vi "Terminal-Alert-6133.vi"(10 "检验次数（5）":i32=5, 11 "6133":T1) -> (3 "6133输出":T1)   [LabVIEW 2014]
uses:
  Terminal-Global-ReferenceValues.vi
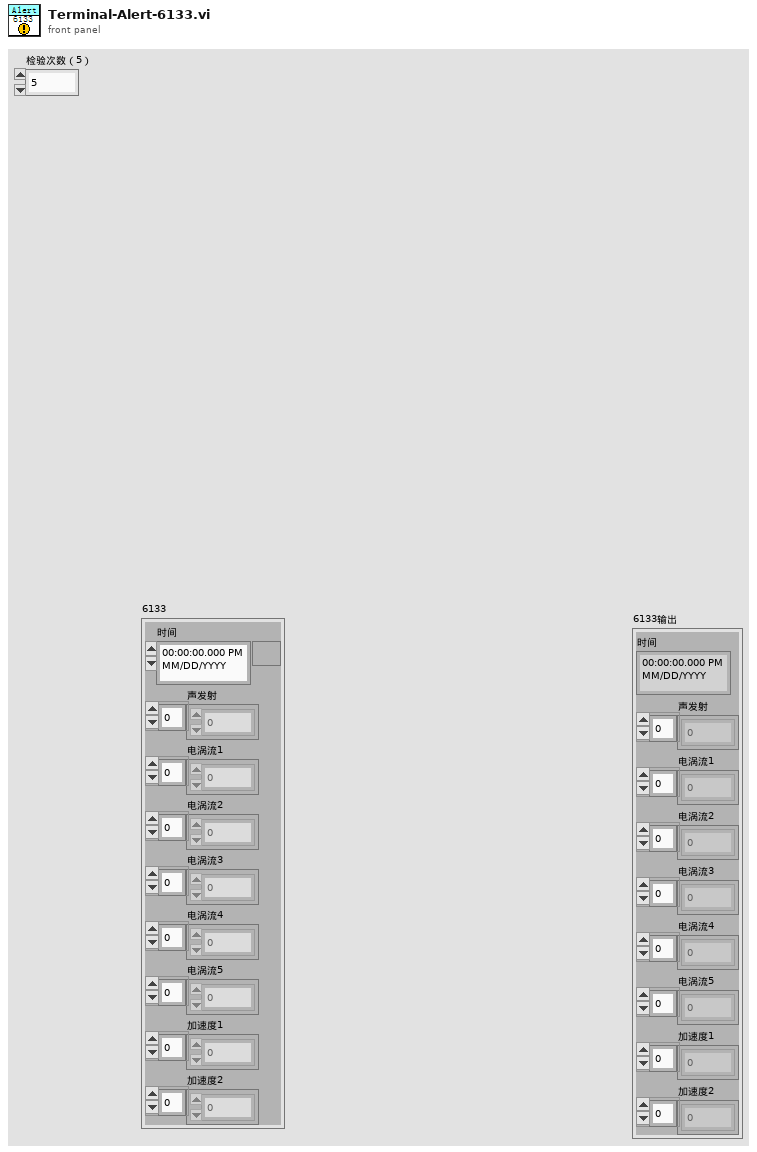
[diagram p1: front panel]
types:
  T1 = cluster{"时间":timestamp, "声发射":sgl[], "电涡流1":sgl[], "电涡流2":sgl[], "电涡流3":sgl[], "电涡流4":sgl[], "电涡流5":sgl[], "加速度1":sgl[], "加速度2":sgl[]}
  T2 = cluster{"试验ID":u32, "报警级别":string, "报警系统":string, "报警详情":string, "备注":string}
  T3 = cluster{"陪试轴承润滑单元":cluster{"出油温度T1":dbl, "出油温度T2":dbl}, "试验轴承润滑单元":cluster{"外壳振动1，A1":dbl, "外壳振动2，A2":dbl, "轴承外圈温度T3":dbl, "出油温度T1":dbl, "摩擦力矩F":dbl, "声发射频率，幅度":dbl}, "加载单元":cluster{"径向油缸力F1'":dbl, "轴向油缸力F2'":dbl}, "主轴监测单元":cluster{"转速W'":dbl, "轴向位移SA":dbl, "径向位移SLR1":dbl, "径向位移SLR2":dbl, "径向位移SRR1":dbl, "径向位移SRR2":dbl}}
  T4 = cluster{"转速W'":dbl, "轴向位移SA":dbl, "径向位移SLR1":dbl, "径向位移SLR2":dbl, "径向位移SRR1":dbl, "径向位移SRR2":dbl}
  T5 = cluster{"外壳振动1，A1":dbl, "外壳振动2，A2":dbl, "轴承外圈温度T3":dbl, "出油温度T1":dbl, "摩擦力矩F":dbl, "声发射频率，幅度":dbl}
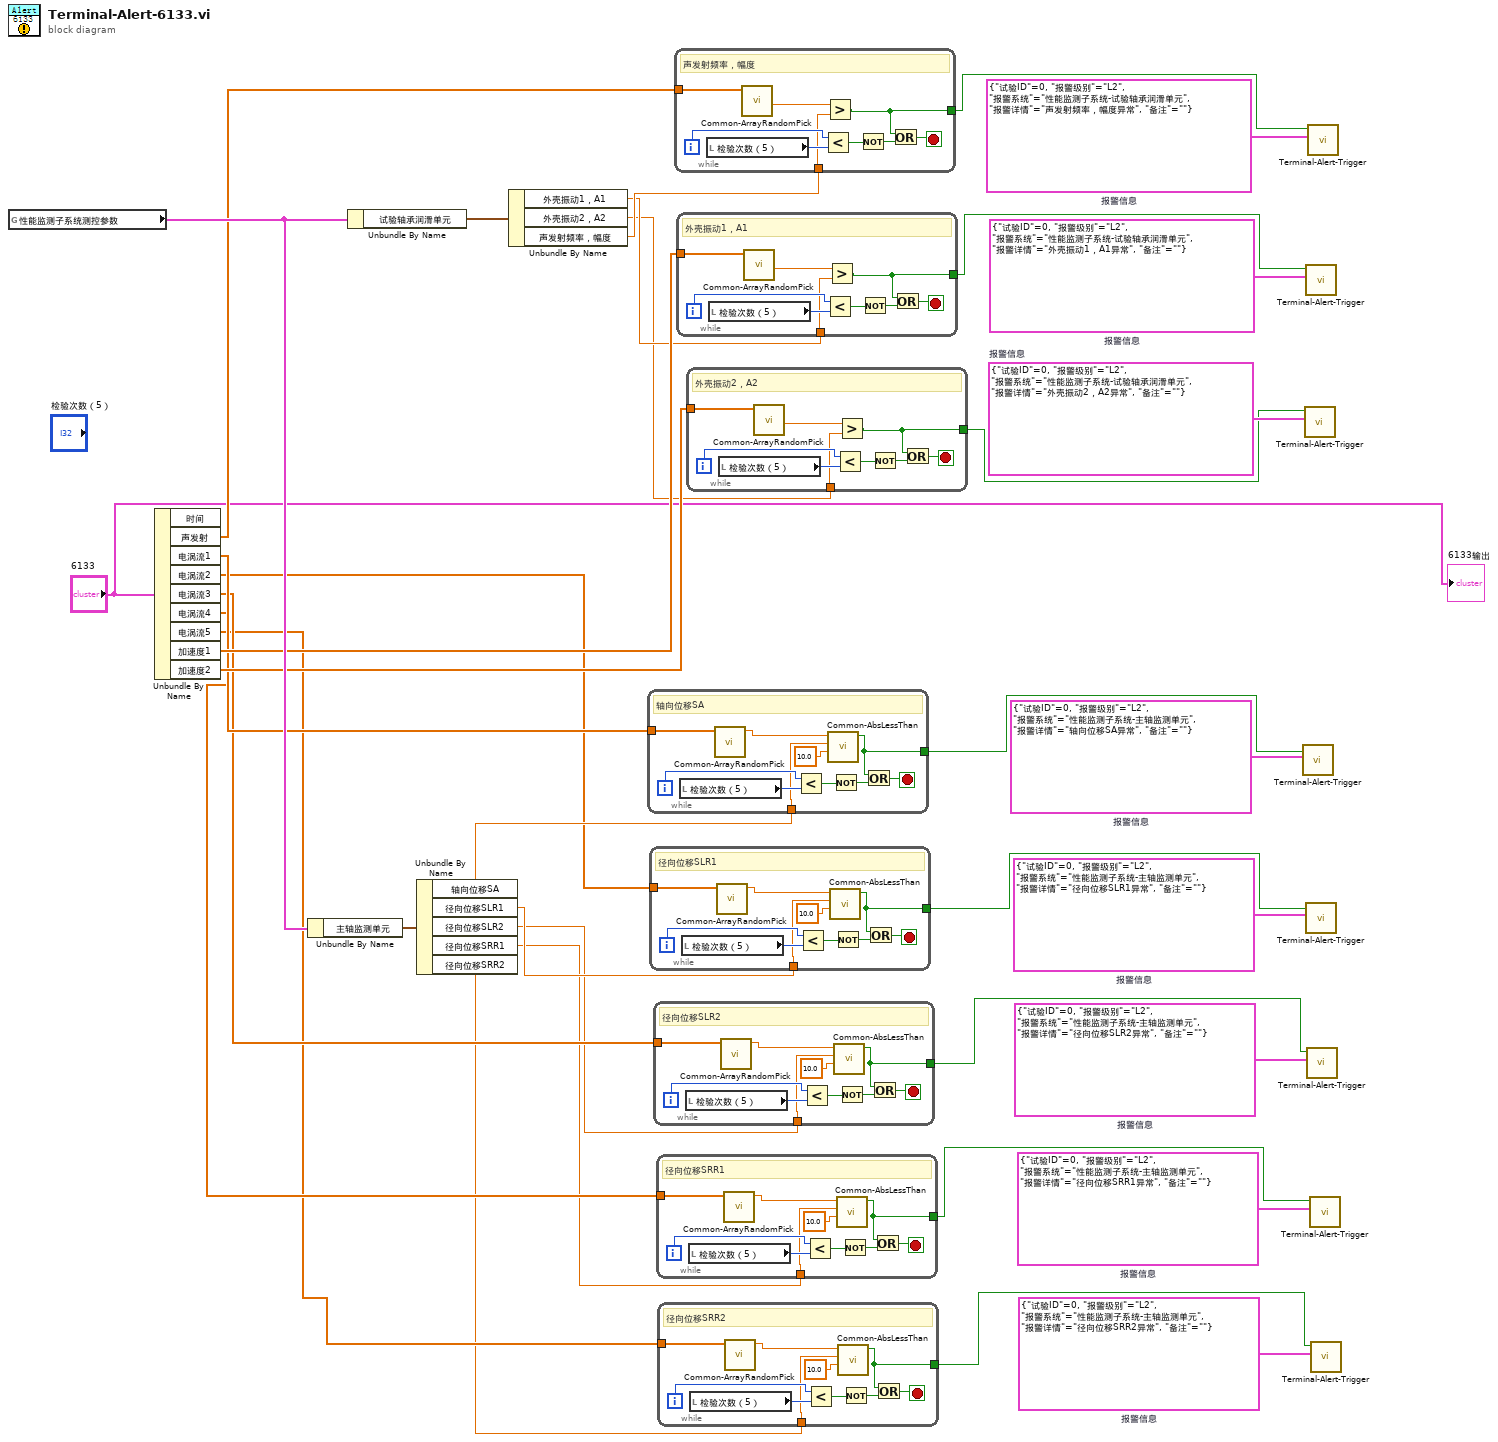
[diagram p0: block diagram]
diagram:
  w27 = T2 {"试验ID"=0, "报警级别"="L2", "报警系统"="性能监测子系统-主轴监测单元", "报警详情"="径向位移SRR2异常", "备注"=""}  # 报警信息
  w26 = T2 {"试验ID"=0, "报警级别"="L2", "报警系统"="性能监测子系统-主轴监测单元", "报警详情"="径向位移SRR1异常", "备注"=""}  # 报警信息
  w28 = T2 {"试验ID"=0, "报警级别"="L2", "报警系统"="性能监测子系统-主轴监测单元", "报警详情"="径向位移SLR2异常", "备注"=""}  # 报警信息
  w29 = T2 {"试验ID"=0, "报警级别"="L2", "报警系统"="性能监测子系统-主轴监测单元", "报警详情"="径向位移SLR1异常", "备注"=""}  # 报警信息
  w30 = T2 {"试验ID"=0, "报警级别"="L2", "报警系统"="性能监测子系统-主轴监测单元", "报警详情"="轴向位移SA异常", "备注"=""}  # 报警信息
  w31 = T2 {"试验ID"=0, "报警级别"="L2", "报警系统"="性能监测子系统-试验轴承润滑单元", "报警详情"="外壳振动2，A2异常", "备注"=""}  # 报警信息
  w33 = T2 {"试验ID"=0, "报警级别"="L2", "报警系统"="性能监测子系统-试验轴承润滑单元", "报警详情"="外壳振动1，A1异常", "备注"=""}  # 报警信息
  w32 = T2 {"试验ID"=0, "报警级别"="L2", "报警系统"="性能监测子系统-试验轴承润滑单元", "报警详情"="声发射频率，幅度异常", "备注"=""}  # 报警信息
  n1 = global read "Terminal-Global-ReferenceValues.vi" "性能监测子系统测控参数"() -> (w35:T3)
  n2 = Unbundle By Name("6133") -> ("声发射"=w25:sgl[], "电涡流1"=w16:sgl[], "电涡流2"=w13:sgl[], "电涡流3"=w12:sgl[], "电涡流4"=w11:sgl[], "电涡流5"=w10:sgl[], "加速度1"=w22:sgl[], "加速度2"=w19:sgl[])  [unwired: 1 out]
  n3 = Unbundle By Name(w35) -> ("主轴监测单元"=w34:T4)
  n4 = Unbundle By Name(w35) -> ("试验轴承润滑单元"=w36:T5)
  n5 = Unbundle By Name(w34) -> ("轴向位移SA"=w14:dbl, "径向位移SLR1"=w9:dbl, "径向位移SLR2"=w8:dbl, "径向位移SRR1"=w7:dbl, "径向位移SRR2"=w6:dbl)
  n6 = Unbundle By Name(w36) -> ("外壳振动1，A1"=w21:dbl, "外壳振动2，A2"=w18:dbl, "声发射频率，幅度"=w24:dbl)
  n7 = while {
    tunnel: w16 -> [w41]
    tunnel: [w40] -> w15
    tunnel: w14 -> [w38]
    i -> [w45]
    stop <- w42 stop-if-true
    # "轴向位移SA"
    n8 = local read "检验次数（5）"() -> (w46:i32)
    n9 = call "Common-ArrayRandomPick.vi"("数组"=w41) -> ("元素"=w39:dbl)  [unwired: 10 in]
    n10 = Less?(x=w45, y=w46) -> (x < y?=w44:bool)
    n11 = call "Common-AbsLessThan.vi"("u"=10.0, "y"=w38, "x"=w39) -> ("abs(x-y) < u?"=w40:bool)  [unwired: 8 in]
    n12 = Not(x=w44) -> (.not. x?=w43:bool)
    n13 = Or(x=w40, y=w43) -> (x .or. y?=w42:bool)
  }
  n14 = while {
    tunnel: w13 -> [w51]
    tunnel: [w50] -> w5
    tunnel: w9 -> [w48]
    i -> [w55]
    stop <- w52 stop-if-true
    # "径向位移SLR1"
    n15 = local read "检验次数（5）"() -> (w56:i32)
    n16 = call "Common-ArrayRandomPick.vi"("数组"=w51) -> ("元素"=w49:dbl)  [unwired: 10 in]
    n17 = Less?(x=w55, y=w56) -> (x < y?=w54:bool)
    n18 = call "Common-AbsLessThan.vi"("u"=10.0, "y"=w48, "x"=w49) -> ("abs(x-y) < u?"=w50:bool)  [unwired: 8 in]
    n19 = Not(x=w54) -> (.not. x?=w53:bool)
    n20 = Or(x=w50, y=w53) -> (x .or. y?=w52:bool)
  }
  n21 = while {
    tunnel: w12 -> [w61]
    tunnel: [w60] -> w4
    tunnel: w8 -> [w58]
    i -> [w65]
    stop <- w62 stop-if-true
    # "径向位移SLR2"
    n22 = local read "检验次数（5）"() -> (w66:i32)
    n23 = call "Common-ArrayRandomPick.vi"("数组"=w61) -> ("元素"=w59:dbl)  [unwired: 10 in]
    n24 = Less?(x=w65, y=w66) -> (x < y?=w64:bool)
    n25 = call "Common-AbsLessThan.vi"("u"=10.0, "y"=w58, "x"=w59) -> ("abs(x-y) < u?"=w60:bool)  [unwired: 8 in]
    n26 = Not(x=w64) -> (.not. x?=w63:bool)
    n27 = Or(x=w60, y=w63) -> (x .or. y?=w62:bool)
  }
  n28 = while {
    tunnel: w11 -> [w71]
    tunnel: [w70] -> w3
    tunnel: w7 -> [w68]
    i -> [w75]
    stop <- w72 stop-if-true
    # "径向位移SRR1"
    n29 = local read "检验次数（5）"() -> (w76:i32)
    n30 = call "Common-ArrayRandomPick.vi"("数组"=w71) -> ("元素"=w69:dbl)  [unwired: 10 in]
    n31 = Less?(x=w75, y=w76) -> (x < y?=w74:bool)
    n32 = call "Common-AbsLessThan.vi"("u"=10.0, "y"=w68, "x"=w69) -> ("abs(x-y) < u?"=w70:bool)  [unwired: 8 in]
    n33 = Not(x=w74) -> (.not. x?=w73:bool)
    n34 = Or(x=w70, y=w73) -> (x .or. y?=w72:bool)
  }
  n35 = while {
    tunnel: w10 -> [w81]
    tunnel: [w80] -> w2
    tunnel: w6 -> [w78]
    i -> [w85]
    stop <- w82 stop-if-true
    # "径向位移SRR2"
    n36 = local read "检验次数（5）"() -> (w86:i32)
    n37 = call "Common-ArrayRandomPick.vi"("数组"=w81) -> ("元素"=w79:dbl)  [unwired: 10 in]
    n38 = Less?(x=w85, y=w86) -> (x < y?=w84:bool)
    n39 = call "Common-AbsLessThan.vi"("u"=10.0, "y"=w78, "x"=w79) -> ("abs(x-y) < u?"=w80:bool)  [unwired: 8 in]
    n40 = Not(x=w84) -> (.not. x?=w83:bool)
    n41 = Or(x=w80, y=w83) -> (x .or. y?=w82:bool)
  }
  n42 = while {
    tunnel: w25 -> [w88]
    tunnel: [w89] -> w23
    tunnel: w24 -> [w90]
    i -> [w94]
    stop <- w91 stop-if-true
    # "声发射频率，幅度"
    n43 = local read "检验次数（5）"() -> (w95:i32)
    n44 = call "Common-ArrayRandomPick.vi"("数组"=w88) -> ("元素"=w87:dbl)  [unwired: 10 in]
    n45 = Less?(x=w94, y=w95) -> (x < y?=w93:bool)
    n46 = Greater?(x=w87, y=w90) -> (0:w89:bool)
    n47 = Not(x=w93) -> (.not. x?=w92:bool)
    n48 = Or(x=w89, y=w92) -> (x .or. y?=w91:bool)
  }
  n49 = while {
    tunnel: w22 -> [w97]
    tunnel: [w98] -> w20
    tunnel: w21 -> [w99]
    i -> [w103]
    stop <- w100 stop-if-true
    # "外壳振动1，A1"
    n50 = local read "检验次数（5）"() -> (w104:i32)
    n51 = call "Common-ArrayRandomPick.vi"("数组"=w97) -> ("元素"=w96:dbl)  [unwired: 10 in]
    n52 = Less?(x=w103, y=w104) -> (x < y?=w102:bool)
    n53 = Greater?(x=w96, y=w99) -> (0:w98:bool)
    n54 = Not(x=w102) -> (.not. x?=w101:bool)
    n55 = Or(x=w98, y=w101) -> (x .or. y?=w100:bool)
  }
  n56 = while {
    tunnel: w19 -> [w106]
    tunnel: [w107] -> w17
    tunnel: w18 -> [w108]
    i -> [w112]
    stop <- w109 stop-if-true
    # "外壳振动2，A2"
    n57 = local read "检验次数（5）"() -> (w113:i32)
    n58 = call "Common-ArrayRandomPick.vi"("数组"=w106) -> ("元素"=w105:dbl)  [unwired: 10 in]
    n59 = Less?(x=w112, y=w113) -> (x < y?=w111:bool)
    n60 = Greater?(x=w105, y=w108) -> (0:w107:bool)
    n61 = Not(x=w111) -> (.not. x?=w110:bool)
    n62 = Or(x=w107, y=w110) -> (x .or. y?=w109:bool)
  }
  n63 = call "Terminal-Alert-Trigger.vi"("报警信息"=w30, "是否触发"=w15) -> ()  [unwired: 9 in, 1 out]
  n64 = call "Terminal-Alert-Trigger.vi"("报警信息"=w31, "是否触发"=w17) -> ()  [unwired: 9 in, 1 out]
  n65 = call "Terminal-Alert-Trigger.vi"("报警信息"=w33, "是否触发"=w20) -> ()  [unwired: 9 in, 1 out]
  n66 = call "Terminal-Alert-Trigger.vi"("报警信息"=w29, "是否触发"=w5) -> ()  [unwired: 9 in, 1 out]
  n67 = call "Terminal-Alert-Trigger.vi"("报警信息"=w28, "是否触发"=w4) -> ()  [unwired: 9 in, 1 out]
  n68 = call "Terminal-Alert-Trigger.vi"("报警信息"=w32, "是否触发"=w23) -> ()  [unwired: 9 in, 1 out]
  n69 = call "Terminal-Alert-Trigger.vi"("报警信息"=w26, "是否触发"=w3) -> ()  [unwired: 9 in, 1 out]
  n70 = call "Terminal-Alert-Trigger.vi"("报警信息"=w27, "是否触发"=w2) -> ()  [unwired: 9 in, 1 out]
  "6133输出" <- "6133"
